vi "Plot Helper (Fixed).vi"(5 "error b vector":dbl[](array[numeric]), 7 "error a vector":dbl[](array[numeric]), 8 "error in (no error)":errorcluster, 9 "y vector":dbl[](array[numeric]), 10 "x vector":dbl[](array[numeric]), 11 "2D Plot Class Obj Array in":refnum<class "2D Plot Datatype.lvclass">[](array[class])) -> (0 "error out":errorcluster, 3 "2D Plot Class Obj Array out":refnum<class "2D Plot Datatype.lvclass">[](array[class]))   [LabVIEW 2017, in "2D Error Bar Datatype.lvclass"]
doc: "Graphs a plot that displays the percentage or vector of error at each point above and below the line graph. Multiple references to this VI generate multiple plots on the same graph."
uses:
  <vilib>/Math Plots/2D Math Plots/2D Error Bar/2D Error Bar Datatype/2D Error Bar Datatype.lvclass
  <vilib>/Math Plots/2D Math Plots/2D Plot/2D Plot Datatype/2D Plot Datatype.lvclass
  e:/builds/penguin/labview/branches/2017/dev/dist/vi.lib/Math Plots/2D Math Plots/2D Plot/2D Plot Datatype/2D Plot Datatype.lvclass
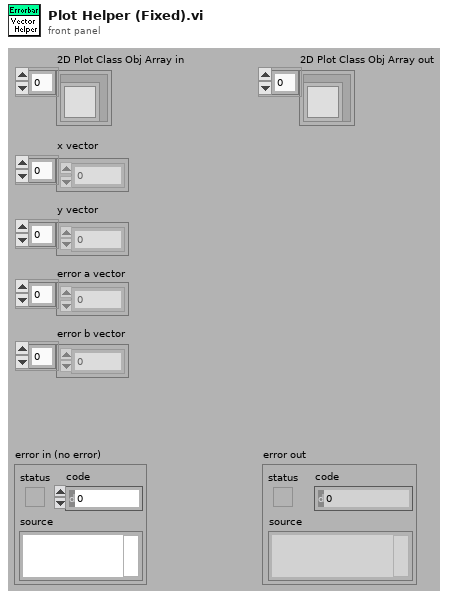
[diagram p1: front panel]
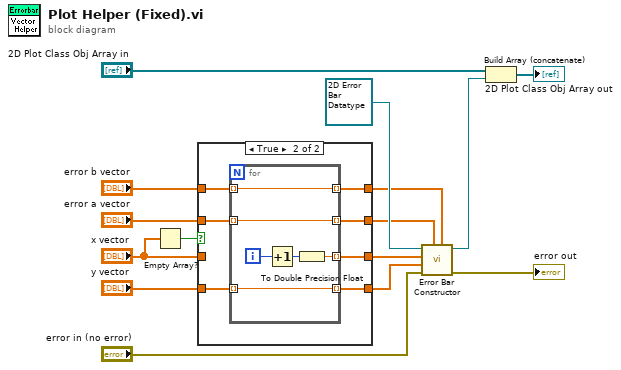
[diagram p0: block diagram]
diagram:
  n1 = Empty Array?(array="x vector") -> (empty?=w1:bool)
  n2 = case shown="True" w1 {
    tunnel: "y vector" -> [w23 w32]
    tunnel: [w22 w28] -> w14
    tunnel: [w21 w29] -> w13
    tunnel: [w20 w30] -> w6
    tunnel: "error a vector" -> [w19 w33]
    tunnel: [w18 w31] -> w4
    tunnel: "error b vector" -> [w17 w34]
    tunnel: "x vector" -> [w16 _]
    frame False {
      n3 = for {
        tunnel: [w27] -> w21 mode=indexing
        tunnel: w16 -> [w27] mode=indexing
        tunnel: [w26] -> w22 mode=indexing
        tunnel: w23 -> [w26] mode=indexing
        tunnel: [w25] -> w20 mode=indexing
        tunnel: w19 -> [w25] mode=indexing
        tunnel: [w24] -> w18 mode=indexing
        tunnel: w17 -> [w24] mode=indexing
      }
    }
    frame True {
      n4 = for {
        tunnel: [w36] -> w29 mode=indexing
        tunnel: [w40] -> w28 mode=indexing
        tunnel: w32 -> [w40] mode=indexing
        tunnel: [w39] -> w30 mode=indexing
        tunnel: w33 -> [w39] mode=indexing
        tunnel: [w38] -> w31 mode=indexing
        tunnel: w34 -> [w38] mode=indexing
        i -> [w37]
        n5 = Increment(x=w37) -> (x+1=w35:i32)
        n6 = To Double Precision Float(number=w35) -> (double precision float=w36:dbl)
      }
    }
  }
  n7 = call <vilib>:"Error Bar Constructor.vi"("error b vector"=w4, "error a vector"=w6, "error in (no error)"="error in (no error)", "y vector"=w14, "x vector"=w13, "2D Error Bar Datatype.lvclass in"=refnum<class "2D Error Bar Datatype.lvclass"> refnum ("3D Quiver Datatype.lvclass in")) -> ("error out"=→"error out":errorcluster, "2D Error Bar Datatype.lvclass out"=w11:refnum<class "2D Error Bar Datatype.lvclass">)  [unwired: 1 in, 3 out]
  n8 = Build Array (concatenate)("2D Plot Class Obj Array in", w11) -> (→"2D Plot Class Obj Array out":refnum<class "2D Plot Datatype.lvclass">[])
